vi "Add Client.vi"(8 "error in (no error)":errorcluster, 9 "Client ID":string, 10 "WebSocket Connection":refnum<k5>, 11 "WebSocket Service Actor in":refnum<class "WebSocket Service.lvclass">) -> (0 "error out":errorcluster, 3 "WebSocket Service Actor out":refnum<class "WebSocket Service.lvclass">)   [LabVIEW 2016, in "WebSocket Actors.lvlib" / "WebSocket Service.lvclass"]
uses:
  WebSocket Service.lvclass
  C:/Program Files (x86)/National Instruments/LabVIEW 2016/vi.lib/ActorFramework/Actor/Actor.lvclass
  WebSocket Connection/WebSocket Connection.lvclass
  WebSocket Service Messages/WebSocket Service Connection Handler Msg/WebSocket Service Connection Handler Msg.lvclass
  C:/Projects/Shared Libraries/WebSocket Actor/WebSocket Actor/Abstract Messages/WebSocket Connection Handler Msg/WebSocket Connection Handler Msg.lvclass
  <vilib>/ActorFramework/Actor/Actor.lvclass/Actor.ctl
  <vilib>/ActorFramework/Message Enqueuer/Message Enqueuer.lvclass/Message Enqueuer.ctl
  WebSocket Service.lvclass/WebSocket Service.ctl
  WebSocket Connection/WebSocket Connection.lvclass/WebSocket Connection.ctl
  WebSocket Connection/properties/Write WebSocket Connection.vi
  WebSocket Connection/properties/Write Peer ID.vi
  <vilib>/ActorFramework/Message Enqueuer/Init from Existing Queue.vi
  WebSocket Connection/properties/Write WebSocket Data Handler.vi
  <vilib>/ActorFramework/Message Enqueuer/Message Enqueuer.lvclass
  <vilib>/ActorFramework/Actor/Actor.lvclass
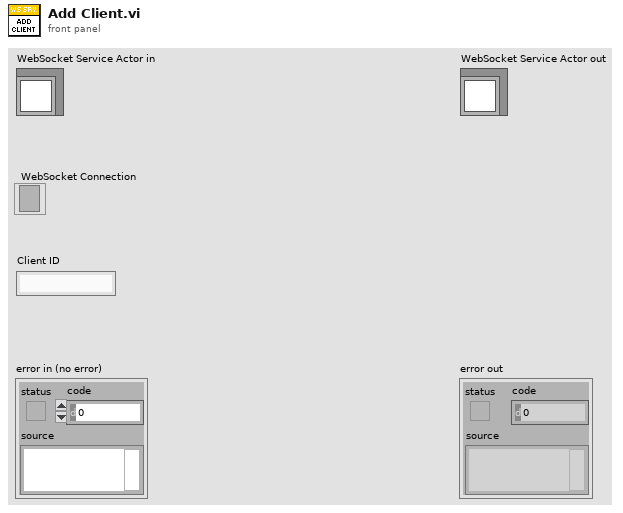
[diagram p1: front panel]
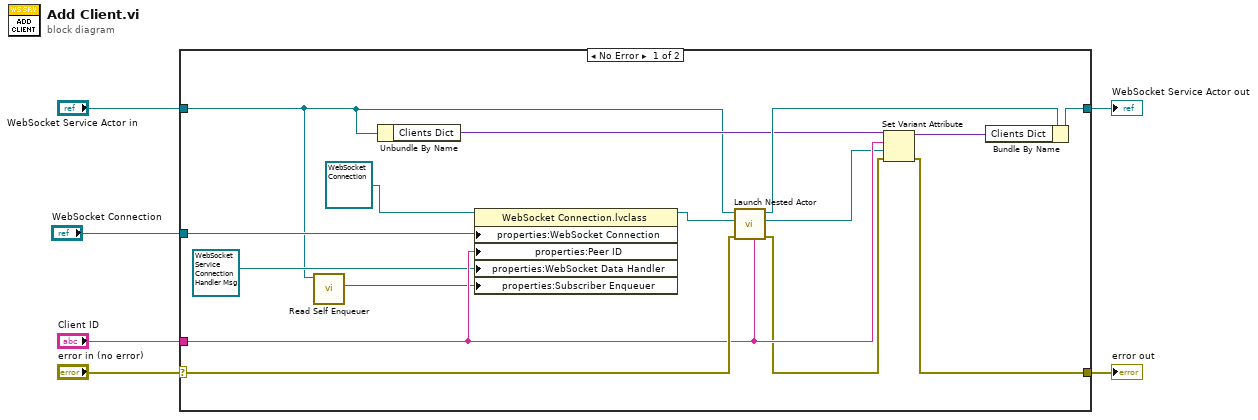
[diagram p0: block diagram]
diagram:
  n1 = case shown="No Error" "error in (no error)" {
    selector: "error in (no error)" -> [w19 w23]
    tunnel: [w10 w23] -> w5
    tunnel: [w16 w22] -> w3
    tunnel: "WebSocket Service Actor in" -> [w8 w22]
    tunnel: "WebSocket Connection" -> [w17 _]
    tunnel: "Client ID" -> [w13 _]
    frame No Error {
      n2 = call <vilib>:"Read Self Enqueuer.vi"("Actor"=w8) -> ("Self Enqueuer"=w7:refnum<class "Message Enqueuer.lvclass">)  [unwired: 10 in]
      n3 = Unbundle By Name(w8) -> ("Clients Dict"=w15:variant)
      n4 = property class="WebSocket Connection.lvclass"(reference=refnum<class "WebSocket Connection.lvclass"> refnum ("WebSocket Connection.lvclass"), "properties:WebSocket Connection"=w17, "properties:Peer ID"=w13, "properties:WebSocket Data Handler"=refnum<class "WebSocket Service Connection Handler Msg.lvclass"> refnum ("WebSocket Actors.lvlib:WebSocket Service Data Handler Msg.lvclass"), "properties:Subscriber Enqueuer"=w7) -> (reference out=w21:refnum<class "WebSocket Connection.lvclass">)  [unwired: 1 in, 1 out]
      n5 = call <vilib>:"Launch Nested Actor.vi"("Debug Alias"=w13, "error in (no error)"=w19, "Nested Actor"=w21, "Caller Actor in"=w8) -> ("error out"=w11:errorcluster, "Nested Actor's Enqueuer"=w12:refnum<class "Message Enqueuer.lvclass">, "Caller Actor out"=w20:refnum<class "WebSocket Service.lvclass">)  [unwired: 5 in]
      n6 = Set Variant Attribute(Variant=w15, name=w13, value=w12, error in=w11) -> (Variant out=w14:variant, error out=w10:errorcluster)  [unwired: 1 out]
      n7 = Bundle By Name(cluster=w20, "Clients Dict"=w14) -> (w16:refnum<class "WebSocket Service.lvclass">)
    }
    frame Error {
    }
  }
  "error out" <- w5
  "WebSocket Service Actor out" <- w3
